vi "small_rand_rotate.vi"(11 "NXT 2":T1={"Hardware"="NXT", "Flattened String"=""}) -> (0 "degrees rotated":dbl, 1 "right(T)/left(F)":bool, 3 "NXT":T1={"Hardware"="NXT", "Flattened String"=""})   [LabVIEW 2012]
uses:
  <vilib>/NXT/Subs/LVHSConnector.ctl
  <vilib>/NXT/Subs/MotorOutput.ctl
  <vilib>/NXT/Dual Mode Library/prims/sign/sign_float.vi
  <vilib>/NXT/Dual Mode Library/Display/drawNumber_float.vi
  <vilib>/NXT/Dual Mode Library/Waits/Wait_Num.vi
  <vilib>/NXT/Dual Mode Library/Motors/MotorBrake.vi
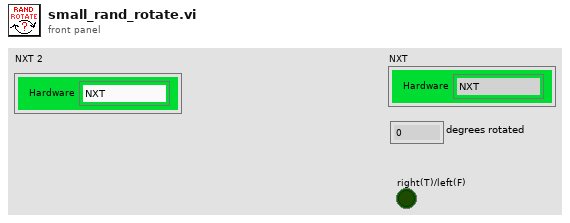
[diagram p1: front panel]
types:
  T1 = typedef "LVHSConnector.ctl" = cluster{"Hardware":string, "Flattened String":string}
  T2 = typedef "MotorOutput.ctl" = u8
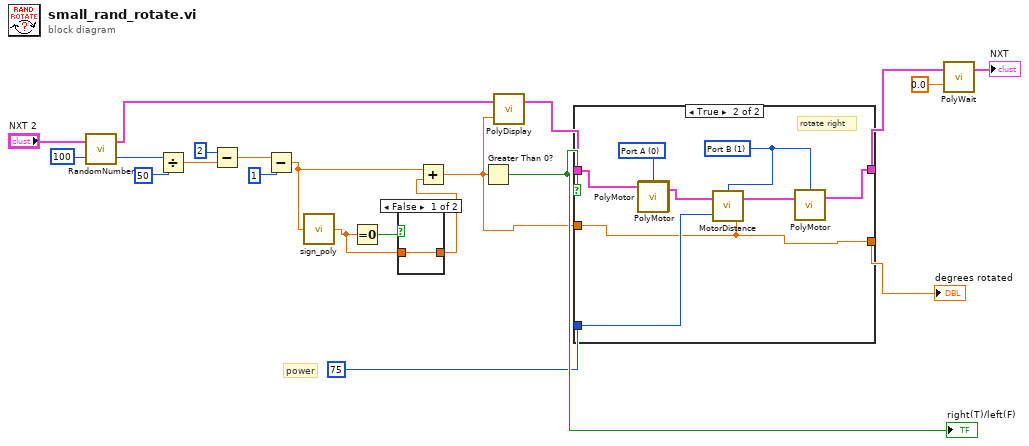
[diagram p0: block diagram]
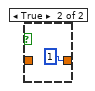
[diagram p2: hidden frame]
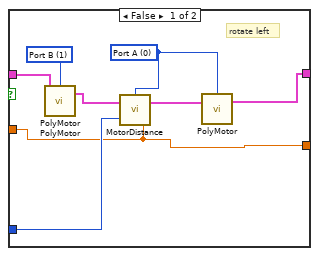
[diagram p3: hidden frame]
diagram:
  # "power"
  n1 = call <vilib>:"RandomNumber.vi"("Max Value"=u16 100, "NXT"="NXT 2") -> ("Random Number"=w8:u16, "NXT"=w9:T1)  [unwired: 1 in]
  n2 = Divide(x=w8, y=u16 50 ("Max Value")) -> (x/y=w6:dbl)
  n3 = Subtract(x=u16 2 ("Max Value"), y=w6) -> (x-y=w17:dbl)
  n4 = Subtract(x=w17, y=u16 1 ("Max Value")) -> (x-y=w4:dbl)
  n5 = call-poly <vilib>:"sign_poly.vi"("number"=w4) -> ("-1, 0, 1"=w2:dbl)  [unwired: 4 in]
  n6 = Equal To 0?(x=w2) -> (x = 0?=w3:bool)
  n7 = case shown="False" w3 {
    tunnel: w2 -> [w22 _]
    tunnel: [w22 u16 1 ("Max Value")] -> w1
    frame False {
    }
    frame True {
    }
  }
  n8 = Add(x=w4, y=w1) -> (x+y=w5:dbl)
  n9 = Greater Than 0?(x=w5) -> (x > 0?=w15:bool)
  "right(T)/left(F)" <- w15
  n10 = call-poly <vilib>:"PolyDisplay.vi"("number"=w5, "NXT"=w9) -> ("NXT"=w13:T1)  [unwired: 2 in]
  n11 = case shown="True" w15 {
    tunnel: w13 -> [w27 w35]
    tunnel: w5 -> [w24 w32]
    tunnel: u16 75 ("Max Value") -> [w26 w34]
    tunnel: [w25 w33] -> w12
    tunnel: [w24 w32] -> w20
    frame False {
      w29 = T2 0 items=["Port A"=0, "Port B"=1, "Port C"=2, "Ports A & B"=4, "Ports A & C"=5, "Ports B & C"=6, "as"=3] ("Output Port (All Ports)")
      w28 = T2 1 items=["Port A"=0, "Port B"=1, "Port C"=2, "Ports A & B"=4, "Ports A & C"=5, "Ports B & C"=6, "as"=3] ("Output Port (All Ports)")
      # "rotate left"
      n12 = call-poly <vilib>:"PolyMotor.vi"("NXT"=w27) -> ()  [unwired: 3 in, 1 out]
      n13 = call-poly <vilib>:"PolyMotor.vi"("Port (All Ports)"=w28) -> ("NXT"=w31:T1)  [unwired: 3 in]
      n14 = call <vilib>:"MotorDistance.vi"("Power (75)"=w26, "Angle of Rotation (360)"=w24, "NXT"=w31, "Output Port (All Ports)"=w29) -> ("NXT"=w30:T1)
      n15 = call-poly <vilib>:"PolyMotor.vi"("NXT"=w30, "Port (All Ports)"=w29) -> ("NXT"=w25:T1)  [unwired: 2 in]
    }
    frame True {
      w37 = T2 1 items=["Port A"=0, "Port B"=1, "Port C"=2, "Ports A & B"=4, "Ports A & C"=5, "Ports B & C"=6, "as"=3] ("Output Port (All Ports)")
      w36 = T2 0 items=["Port A"=0, "Port B"=1, "Port C"=2, "Ports A & B"=4, "Ports A & C"=5, "Ports B & C"=6, "as"=3] ("Output Port (All Ports)")
      # "rotate right"
      n16 = call-poly <vilib>:"PolyMotor.vi"("Port (All Ports)"=w36) -> ("NXT"=w39:T1)  [unwired: 3 in]
      n17 = call-poly <vilib>:"PolyMotor.vi"("NXT"=w35) -> ()  [unwired: 3 in, 1 out]
      n18 = call <vilib>:"MotorDistance.vi"("Power (75)"=w34, "Angle of Rotation (360)"=w32, "NXT"=w39, "Output Port (All Ports)"=w37) -> ("NXT"=w38:T1)
      n19 = call-poly <vilib>:"PolyMotor.vi"("NXT"=w38, "Port (All Ports)"=w37) -> ("NXT"=w33:T1)  [unwired: 2 in]
    }
  }
  "degrees rotated" <- w20
  n20 = call-poly <vilib>:"PolyWait.vi"("Time (1 sec)"=sgl 0.0, "NXT"=w12) -> ("NXT"=→"NXT":T1)  [unwired: 2 in]
